vi "Pit Scouting.vi"() -> ()   [LabVIEW 2013]
panel:
  in  "What Mechanisims Do They Pick Up With?":string
  in  "Did They Do Autonomous, If So, How?":string
  in  "Can They Pick Up Trash Cans?":string(combo)
  in  "How Do They Pick Up Trash Cans?":string
  in  "How Do They Pick Up Totes?":string
  in  "Cooperation With Team?":string
  in  "Perfered Starting Position?":string
  in  "Starting Position On Field?":string
  in  "Can They Move Litter?":string(combo)
  in  "Do Human Players Throw Litter?":string(combo)
  in  "Can They Put Them In a Trash Can?":string(combo)
  in  "Can They Pick Up Noodles?":string(combo)
  in  "Max Stack Height?":string(combo)
  in  "How Many Totes Can They Move?":string(combo)
  in  "What Drive Train Did They Use?":string
  in  "What Wheels Did They Use?":string
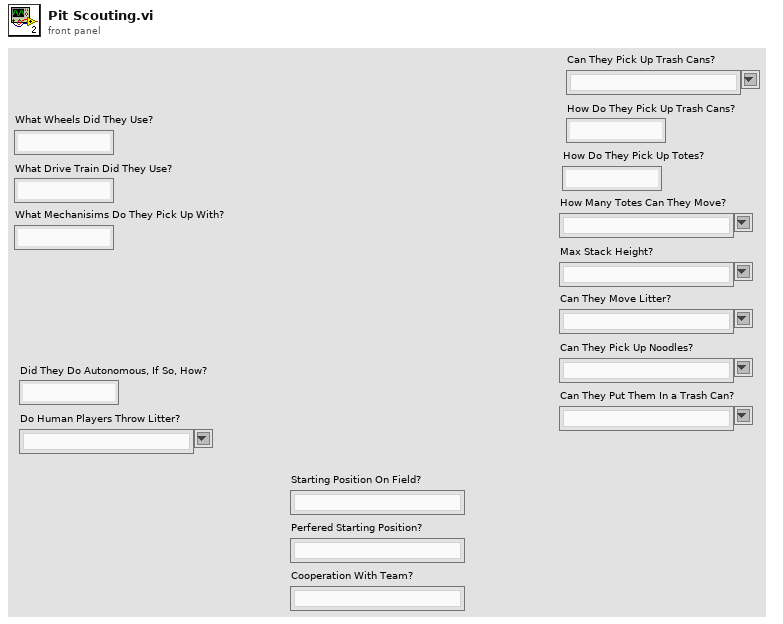
[diagram p1: front panel]
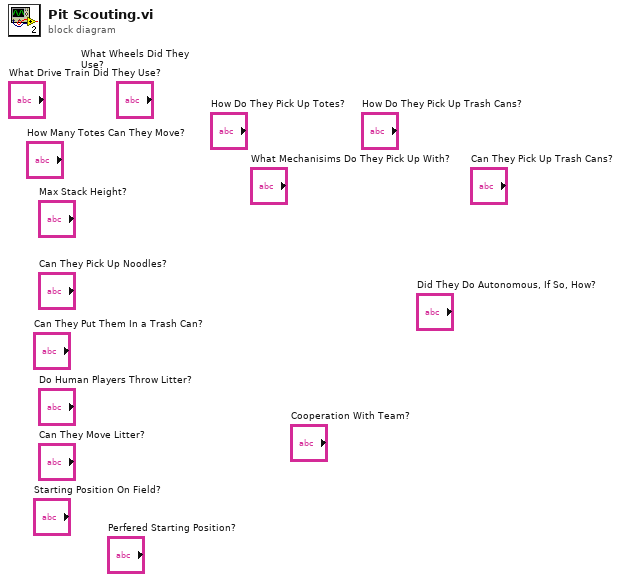
[diagram p0: block diagram]
diagram:
